vi "Read_Image_Dataset.vi"(7 "Labels":string[](array[string]), 8 "error in (no error)":errorcluster, 11 "Image File Paths":path[](array[path])) -> (0 "error out":errorcluster, 3 "Dataset Out":T1={"Inputs Ref."=variant(refnum<data-value> refnum), "Outputs Ref."=refnum, "Dataset_Size"=0, "Dims_In"={"C"=0, "H"=0, "W"=0}, "Dims_Out"=0, "Labels"=[], "File Paths"=[], "Custom_Data"=variant})   [LabVIEW 2020]
uses:
  <vilib>/Ngene/Deep Learning Toolkit/Toolkit/NN_Data/API/DataSet/DataSet_Types/NN_DataSet(In3D_Out1D).ctl
  <vilib>/Ngene/Deep Learning Toolkit/Toolkit/NN_Data/Controls/DataRef_Types/2D/NN_Data_ref(2D_SGL).ctl
  <vilib>/Ngene/Deep Learning Toolkit/Toolkit/NN_Data/API/NN_Dims(C,H,W).ctl
  <vilib>/Ngene/Deep Learning Toolkit/Toolkit/Deep_Learning_Toolkit_by_Ngene.lvlib
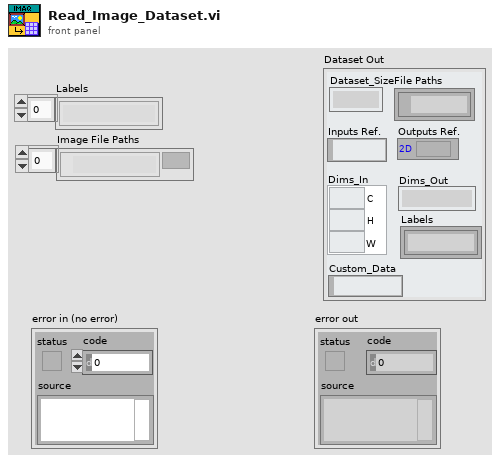
[diagram p1: front panel]
types:
  T1 = typedef "Deep_Learning_Toolkit_by_Ngene.lvlib/NN_DataSet(In3D_Out1D).ctl" = cluster{"Inputs Ref.":variant, "Outputs Ref.":T2, "Dataset_Size":i32, "Dims_In":T3, "Dims_Out":i32, "Labels":string[], "File Paths":path[], "Custom_Data":variant}
  T2 = typedef "Deep_Learning_Toolkit_by_Ngene.lvlib/NN_Data_ref(2D_SGL).ctl" = refnum<data-value>
  T3 = typedef "Deep_Learning_Toolkit_by_Ngene.lvlib/NN_Dims(C,H,W).ctl" = cluster{"C":i32, "H":i32, "W":i32}
  T4 = typedef "Image Type" = u32
  T5 = typedef "IMAQ Image.ctl" = refnum<image>
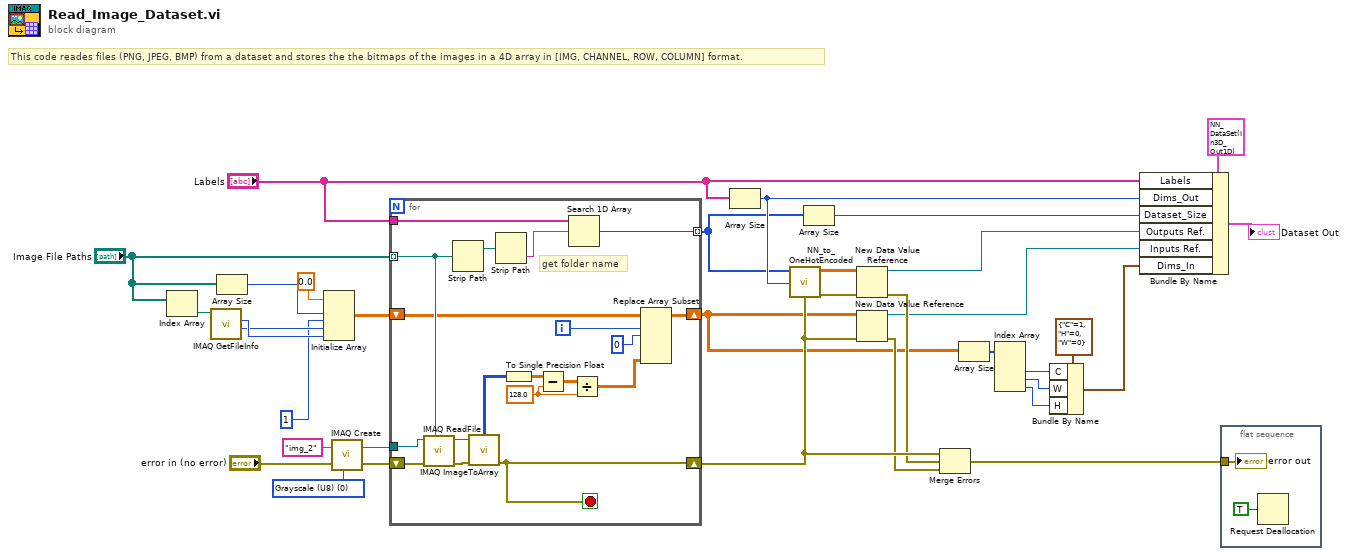
[diagram p0: block diagram]
diagram:
  w30 = T4 0 items=["Grayscale (U8)", "Grayscale (I16)", "Grayscale (SGL)", "Complex (CSG)", "RGB (U32)", "HSL (U32)", "RGB (U64)", "Grayscale (U16)"] ("Image Type")
  # "This code reades files (PNG, JPEG, BMP) from a dataset and stores the the bitmaps of the images in a 4D array in [IMG, CHANNEL, ROW, COLUMN] format."
  n1 = Index Array(array="Image File Paths") -> (element=w15:path)  [unwired: 1 in]
  n2 = call "IMAQ GetFileInfo"("File Path"=w15) -> ("Y Resolution"=w13:i32, "X Resolution"=w14:i32)  [unwired: 4 in, 5 out]
  n3 = Array Size(array="Image File Paths") -> (size(s)=w12:i32)
  n4 = Initialize Array(sgl 0.0 ("y"), w12, 1 ("dimension size"), w13, w14) -> (w9:sgl[][][][])
  n5 = call "IMAQ Create"("Image Name"="img_2", "Image Type"=w30, "error in (no error)"="error in (no error)") -> ("New Image"=w31:T5, "error out"=w28:errorcluster)  [unwired: 2 in]
  n6 = for {
    tunnel: "Image File Paths" -> [w51] mode=indexing
    tunnel: [w45] -> w20 mode=indexing
    tunnel: w31 -> [w50]
    tunnel: "Labels" -> [w44]
    shift-right: [w43] -> w23
    shift-left: w28 -> [w47]
    shift-right: [w37] -> w8
    shift-left: w9 -> [w38]
    i -> [w35]
    stop <- w43 stop-if-true
    w39 = sgl 128.0 ("y")
    # "get folder name"
    n7 = call "IMAQ ReadFile"("File Path"=w51, "error in (no error)"=w47, "Image"=w50) -> ("error out"=w49:errorcluster, "Image Out"=w48:T5)  [unwired: 4 in, 3 out]
    n8 = Strip Path(path=w51) -> (stripped path=w52:path)  [unwired: 1 out]
    n9 = call "IMAQ ImageToArray"("error in (no error)"=w49, "Image"=w48) -> ("error out"=w43:errorcluster, "Image Pixels (U8)"=w42:u8[][])  [unwired: 2 in, 3 out]
    n10 = Strip Path(path=w52) -> (name=w46:string)  [unwired: 1 out]
    n11 = To Single Precision Float(number=w42) -> (single precision float=w41:sgl[][])
    n12 = Subtract(x=w41, y=w39) -> (x-y=w40:sgl[][])
    n13 = Search 1D Array(1D array=w44, element=w46) -> (index of element=w45:i32)  [unwired: 1 in]
    n14 = Divide(x=w40, y=w39) -> (x/y=w36:sgl[][])
    n15 = Replace Array Subset(array=w38, new element=w36, index (dim 0)=w35, index (dim 1)=0 ("disabled index (page)")) -> (w37:sgl[][][][])  [unwired: 2 in]
  }
  n16 = Array Size(array="Labels") -> (size(s)=w25:i32)
  n17 = call <vilib>:"NN_to_OneHotEncoded.vi"("Number_of_Labels(-1)"=w25, "Label_Idx"=w20) -> ("Prediction"=w24:sgl[][])  [unwired: 9 in]
  n18 = Array Size(array=w20) -> (size(s)=w19:i32)
  n19 = New Data Value Reference(data value=w24, error in=w23) -> (data value reference=w2:refnum<data-value>, error out=w17:errorcluster)
  n20 = New Data Value Reference(data value=w8, error in=w23) -> (data value reference=w3:refnum<data-value>, error out=w18:errorcluster)
  n21 = Merge Errors(w23, w17, w18) -> (w22:errorcluster)
  n22 = Array Size(array=w8) -> (size(s)=w7:i32[])
  n23 = Index Array(array=w7) -> (element #2=w6:i32, element #3=w5:i32, element #4=w4:i32)  [unwired: 4 in, 1 out]
  n24 = Bundle By Name(cluster=T3 {"C"=1, "H"=0, "W"=0} ("Dims"), "C"=w6, "W"=w5, "H"=w4) -> (w21:T3)
  n25 = Bundle By Name(cluster=T1 {"Inputs Ref."=variant(refnum<data-value> refnum), "Outputs Ref."=refnum, "Dataset_Size"=0, "Dims_In"={"C"=0, "H"=0, "W"=0}, "Dims_Out"=0, "Labels"=[], "File Paths"=[], "Custom_Data"=variant} ("Dataset Refs. (In3D_Out1D)"), "Labels"="Labels", "Dims_Out"=w25, "Dataset_Size"=w19, "Outputs Ref."=w2, "Inputs Ref."=w3, "Dims_In"=w21) -> (→"Dataset Out":T1)
  n26 = flat-sequence {
    tunnel: w22 -> [w53]
    frame #0 {
      n27 = Request Deallocation(TRUE ("flag")) -> ()
      "error out" <- w53
    }
  }
